vi "PLCtoGUI32bit.vi"(9 "DB Val Qty":u16, 11 "DB Input Vals":u8[](array[numeric])=[0, 0, 0, 0]) -> (3 "RealValue":sgl[](array[numeric]))   [LabVIEW 2023]
panel:
  out "Array":bool[](array[boolean])
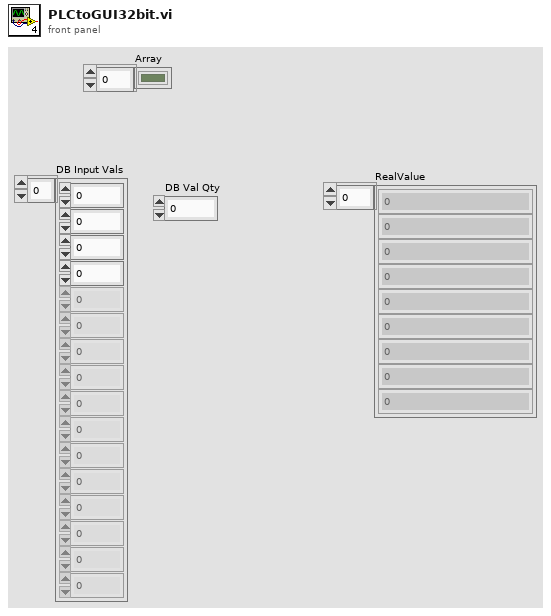
[diagram p1: front panel]
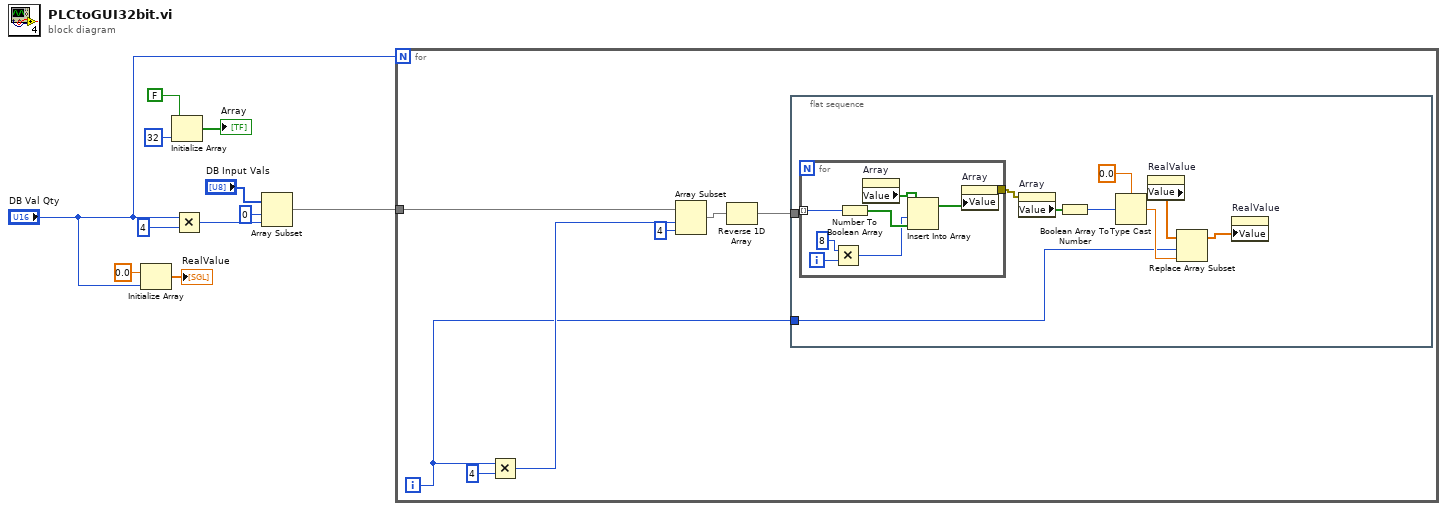
[diagram p0: block diagram]
diagram:
  n1 = Initialize Array(0.0 ("element"), "DB Val Qty") -> (→"RealValue":dbl[])
  n2 = Initialize Array(FALSE, 32 ("dimension size")) -> (→"Array":bool[])
  n3 = Multiply(x="DB Val Qty", y=u8 4) -> (x*y=w6:u16)
  n4 = Array Subset(array="DB Input Vals", index=0, length=w6) -> (w8:u8[])
  n5 = for {
    N: "DB Val Qty" -> [_]
    tunnel: w8 -> [w17]
    i -> [w12]
    n6 = Multiply(x=w12, y=4) -> (x*y=w16:i32)
    n7 = Array Subset(array=w17, index=w16, length=4) -> (w13:u8[])
    n8 = Reverse 1D Array(array=w13) -> (reversed array=w14:u8[])
    n9 = flat-sequence {
      tunnel: w14 -> [w27]
      tunnel: w12 -> [w20]
      frame #0 {
        n10 = for {
          tunnel: w27 -> [w33] mode=indexing
          tunnel: [w28] -> w19
          i -> [w31]
          n11 = Multiply(x=8, y=w31) -> (x*y=w29:i32)
          n12 = Number To Boolean Array(number=w33) -> (Boolean array=w34:bool[])
          n13 = property on="Array" class="Arr (strict)"() -> ("Value"=w35:bool[])  [unwired: 2 in, 2 out]
          n14 = Insert Into Array(array=w35, index=w29, new element=w34) -> (w32:bool[])
          n15 = property on="Array" class="Arr (strict)"("Value"=w32) -> (error out=w28:errorcluster)  [unwired: 2 in, 1 out]
        }
        n16 = property on="Array" class="Arr (strict)"(error in=w19) -> ("Value"=w22:bool[])  [unwired: 1 in, 2 out]
        n17 = Boolean Array To Number(Boolean array=w22) -> (number=w23:u32)
        n18 = Type Cast(type=sgl 0.0, x=w23) -> (*(type *) &x=w24:sgl)
        n19 = property on="RealValue" class="Arr (strict)"() -> ("Value"=w25:sgl[])  [unwired: 2 in, 2 out]
        n20 = Replace Array Subset(array=w25, new element=w24, index=w20) -> (w26:sgl[])
        n21 = property on="RealValue" class="Arr (strict)"("Value"=w26) -> ()  [unwired: 2 in, 2 out]
      }
    }
  }
